vi "转换需保存的状态.vi"(2 "Container State":T1 caption="容器状态", 3 "Display State":T2={"功能选择"=enum."扫描", "数据库引用"=refnum, "扫描参数"={"+ V"=1.0, "+ Δ V"=0.01, "+ limit I"=0.01, "- V"=1.0, "- Δ V"=0.01, "- limit I"=0.01, "NPLC"=1.0, "模型"=FALSE}, "保持时间"={"V"=0.1, "limit I"=0.01, "T"=10000.0, "ΔT"=1.0, "NPLC"=1.0}, "脉冲1"={"t0"=timestamp(0 s since 1904-01-01), "dt"=1.0, "Y"=[]}, "脉冲2"={"t0"=timestamp(0 s since 1904-01-01), "dt"=1.0, "Y"=[]}, "高速脉冲1"={"t0"=timestamp(0 s since 1904-01-01), "dt"=1.0, "Y"=[]}, "高速脉冲2"={"t0"=timestamp(0 s since 1904-01-01), "dt"=1.0, "Y"=[]}, "任意波形"={"t0"=timestamp(0 s since 1904-01-01), "dt"=1.0, "Y"=[]}} caption="显示状态" {"保持时间"."ΔT" min=0.5 max=100.0 step=0.1 format="%#_6ps"; "保持时间"."T" min=10.0 max=4294000.0 step=1.0 format="%#_6ps"; "保持时间"."NPLC" min=1.0 max=20.0 step=1.0; "保持时间"."limit I" min=1e-08 max=3.0 format="%#_6pA"; "保持时间"."V" min=-40.0 max=40.0 format="%#_6pV"; "扫描参数"."NPLC" min=0.001 max=25.0 step=0.001; "扫描参数"."- Δ V" min=5e-05 max=1.0 step=5e-05 format="%#_6pV"; "扫描参数"."+ Δ V" min=5e-05 max=1.0 step=5e-05 format="%#_6pV"; "扫描参数"."- V" min=-40.0 max=40.0 format="%#_6pV"; "扫描参数"."- limit I" min=1e-08 max=3.0 format="%#_6pA"; "扫描参数"."+ limit I" min=1e-08 max=3.0 format="%#_6pA"; "扫描参数"."+ V" min=-40.0 max=40.0 format="%#_6pV"}) -> (1 "Display State To Save":variant caption="待保存显示状态")   [LabVIEW 2020, in "功能选择.xctl"]
uses:
  <vilib>/addons/database/Connection.llb/Conn ObjectReference.ctl
  <vilib>/_xctls/Container State.ctl
  <vilib>/_xctls/XControlSupport.lvlib
  <vilib>/addons/database/NI_Database_API.lvlib
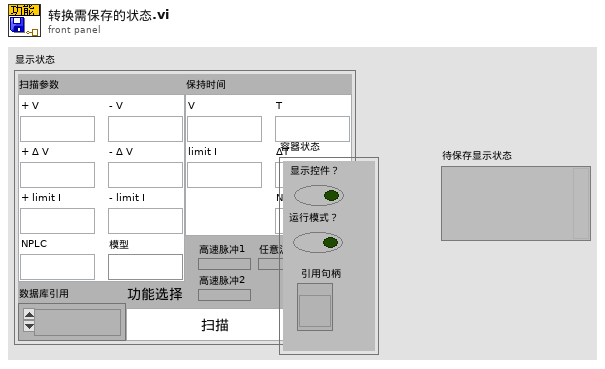
[diagram p1: front panel]
types:
  T1 = typedef "XControlSupport.lvlib/Container State.ctl" = cluster{"Indicator?":bool, "Run Mode?":bool, " Refnum":refnum<vi>}
  T2 = typedef "功能选择.xctl/状态.ctl" = cluster{"功能选择":T3, "数据库引用":T4, "扫描参数":T5, "保持时间":T6, "脉冲1":waveform(dbl), "脉冲2":waveform(dbl), "高速脉冲1":waveform(dbl), "高速脉冲2":waveform(dbl), "任意波形":waveform(dbl)}
  T3 = typedef "功能选择.xctl/功能类型选择.ctl" = enum16{"扫描", "保持时间", "脉冲", "高速脉冲", "任意波形"}
  T4 = typedef "NI_Database_API.lvlib/Conn ObjectReference.ctl" = refnum<k1>
  T5 = typedef "功能选择.xctl/扫描参数.ctl" = cluster{"+ V":dbl, "+ Δ V":dbl, "+ limit I":dbl, "- V":dbl, "- Δ V":dbl, "- limit I":dbl, "NPLC":dbl, "模型":bool}
  T6 = typedef "功能选择.xctl/保持时间.ctl" = cluster{"V":dbl, "limit I":dbl, "T":dbl, "ΔT":dbl, "NPLC":dbl}
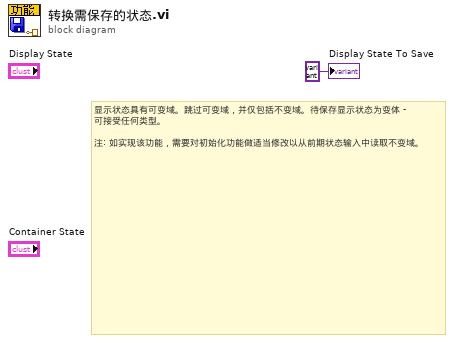
[diagram p0: block diagram]
diagram:
  # "显示状态具有可变域。跳过可变域，并仅包括不变域。待保存显示状态为变体 - 可接受任何类型。\n\n注: 如实现该功能，需要对初始化功能做适当修改以从前期状态输入中读取不变域。"
  "Display State To Save" <- variant ("Display State To Save")
